vi "LeavePOut.vi"(6 "Groups":string[][](array[string]), 8 "error in (no error)":errorcluster caption="entrée d'erreur (pas d'erreur)", 9 "y":string[][](array[string]), 10 "X":string[][](array[string]), 11 "LeavePOut":cluster{"p":i32}={"p"=2}) -> (0 "error out":errorcluster caption="sortie d'erreur", 3 "Split":T1(array[cluster]))   [LabVIEW 2020]
doc: "Leave-P-Out cross-validator\n\nProvides train/test indices to split data in train/test sets. This results in testing on all distinct samples of size p, while the remaining n - p samples form the training set in each iteration.\n\nNote: LeavePOut(p) is NOT equivalent to KFold(n_splits=n_samples // p) which creates non-overlapping test sets.\n\nDue to the high number of iterations which grows combinatorically with the number of samples this cross-validation method can be very costly. For large datasets one should favor KFold, StratifiedKFold or ShuffleSplit.\n\nParameters :\n\n- p : int\nSize of the test sets. Must be strictly less than the number of samples.\n\n\nMethods : Split \n\nGenerate indices to split data into training and test set.\n\nParameters : \n\n- X : array-like of shape (n_samples, n_features)\nTraining data, where n_samples is the number of samples and n_features is the number of features.\n\n- y : array-like of shape (n_samples,)\nThe target variable for supervised learning problems.\n\n- groups : array-like of shape (n_samples,), default=None\nGroup labels for the samples used while splitting the dataset into train/test set.\n\nYields : \n\n- train : ndarray\nThe training set indices for that split.\n\n- test : ndarray\nThe testing set indices for that split."
uses:
  LeavePOut.lvclass
panel:
  out "LeavePOut.lvclass":refnum<class "LeavePOut.lvclass">
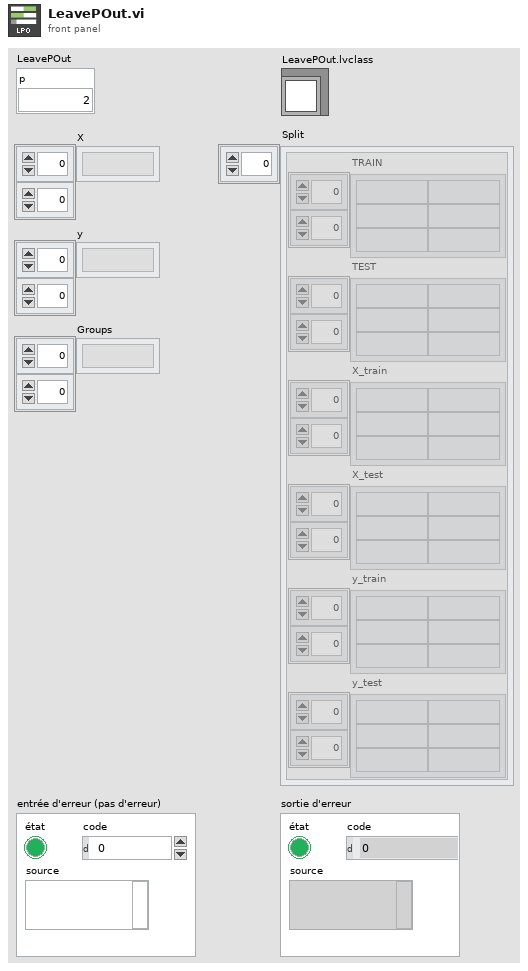
[diagram p1: front panel]
types:
  T1 = cluster{"TRAIN":string[][], "TEST":string[][], "X_train":string[][], "X_test":string[][], "y_train":string[][], "y_test":string[][]}[]
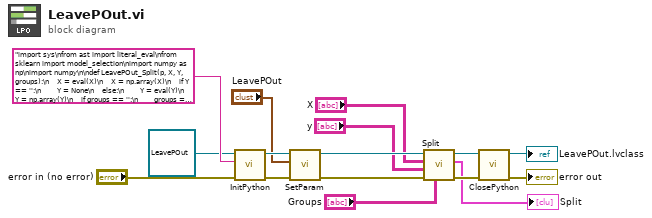
[diagram p0: block diagram]
diagram:
  n1 = call-dynamic "InitPython.vi"("error in (no error)"="error in (no error)", "Python Instruction"="import sys\nfrom ast import literal_eval\nfrom sklearn import model_selection\nimport numpy as np\nimport numpy\n\ndef LeavePOut_Split(p, X, Y, groups):\n    X = eval(X)\n    X = np.array(X)\n    if Y == '':\n        Y = None\n    else:\n        Y = eval(Y)\n        Y = np.array(Y)\n    if groups == '':\n        groups = None\n    else:\n        groups = eval(groups)\n        groups = np.array(groups)\n    list_return = []\n    try:\n        for train_index, test_index in model_selection.LeavePOut(p).split(X, Y, groups):\n            list_return = list_return +[\"TRAIN:\", train_index.tolist(), \"TEST:\", test_index.tolist()]\n            X_train, X_test = X[train_index].tolist(), X[test_index].tolist()\n            y_train, y_test = Y[train_index].tolist(), Y[test_index].tolist()\n            list_return = list_return +[\"X_train:\", X_train, \"X_test:\", X_test, \"y_train:\", y_train, \"y_test:\", y_test]\n        return str(list_return)\n    except:\n        erreur = sys.exc_info()\n        typerr = u\"%s\" % (erreur[0])\n        typerr = typerr[typerr.find(\"'\")+1:typerr.rfind(\"'\")]\n        msgerr = u\"%s\" % (erreur[1])\n        message = str('/!\\\\ {0} : {1}'. format(typerr,msgerr))\n        return message", "Scikit-learn en entrée"=refnum<class "LeavePOut.lvclass"> refnum ("LeavePOut.lvclass")) -> ("error out"=w13:errorcluster, "Scikit-learn en sortie"=w12:refnum<class "LeavePOut.lvclass">)  [unwired: 7 in]
  n2 = call-dynamic "SetParam.vi"("error in (no error)"=w13, "LeavePOut"="LeavePOut", "LeavePOut.lvclass"=w12) -> ("error out"=w10:errorcluster, "LeavePOut.lvclass"=w9:refnum<class "LeavePOut.lvclass">)  [unwired: 7 in]
  n3 = call-dynamic "Split.vi"("Groups"="Groups", "error in (no error)"=w10, "y"="y", "X"="X", "LeavePOut.lvclass"=w9) -> ("error out"=w8:errorcluster, "Split"=→"Split":T1, "LeavePOut.lvclass"=w7:refnum<class "LeavePOut.lvclass">)  [unwired: 4 in]
  n4 = call-dynamic "ClosePython.vi"("error in (no error)"=w8, "Scikit-learn en entrée"=w7) -> ("error out"=→"error out":errorcluster, "Scikit-learn en sortie"=→"LeavePOut.lvclass":refnum<class "LeavePOut.lvclass">)  [unwired: 8 in]
